vi "Identity整体图.vi"() -> ()   [LabVIEW 2014]
panel:
  in  "Identify":bool
  in  "Generate":bool
  in  "Export":bool
  in  "Encrypt":bool
  in  "Decrypt":bool
  in  "Users":bool
  in  "Terminal":bool
  in  "Sign":bool
  in  "Show":bool
  in  "Register":bool
  in  "Personal":bool
  in  "Password":bool
  in  "Log":bool
  in  "Keys":bool
  in  "Key":bool
  in  "Info":bool
  in  "Import":bool
  in  "Identity":bool
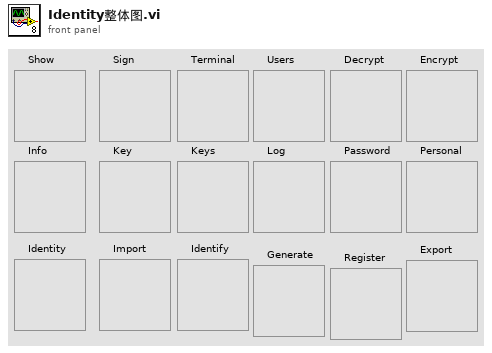
[diagram p1: front panel]
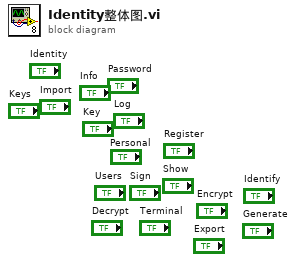
[diagram p0: block diagram]
diagram:
